vi "SET_CAPACITOR.vi"(0 "Arduino Resource in":T3, 1 "Capacitor":dbl=0.8 min=0.0 max=408.8 step=0.8 format="%.1f uF") -> (7 "Arduino Resource out":T3, 10 "error out":errorcluster)   [LabVIEW 2015]
uses:
  <vilib>/LabVIEW Interface for Arduino/Type Defs/Board Type.ctl
  <vilib>/LabVIEW Interface for Arduino/Type Defs/Connection Type.ctl
  <vilib>/LabVIEW Interface for Arduino/LabVIEW Interface for Arduino.lvlib
panel:
  in  "0, 1":i16[](array[numeric])=[1, 1, 1, 1, 1, 1, 1, 1, 1, 1, 1, 1, 1, 1, 1, 1]
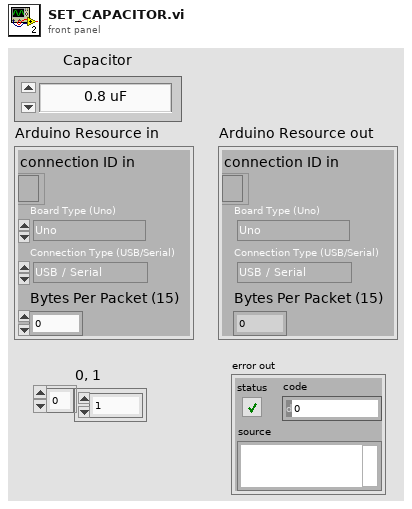
[diagram p1: front panel]
types:
  T1 = typedef "LabVIEW Interface for Arduino.lvlib/Board Type.ctl" = enum16{"Uno", "Dimuelanove w/Atmega 328", "Mega 2560"}
  T2 = typedef "LabVIEW Interface for Arduino.lvlib/Connection Type.ctl" = enum8{"USB / Serial", "XBEE", "BlueSmirf (Bluetooth)"}
  T3 = cluster{"connection ID in":refnum<k31>, "Board Type (Uno)":T1, "Connection Type (USB/Serial)":T2, "Bytes Per Packet (15)":u32}
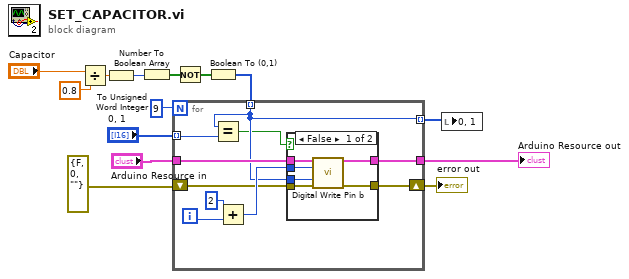
[diagram p0: block diagram]
diagram:
  n1 = Divide(x="Capacitor", y=0.8) -> (x/y=w10:dbl)
  n2 = To Unsigned Word Integer(number=w10) -> (unsigned 16bit integer=w13:u16)
  n3 = Number To Boolean Array(number=w13) -> (Boolean array=w9:bool[])
  n4 = Not(x=w9) -> (.not. x?=w8:bool[])
  n5 = Boolean To (0,1)(Boolean=w8) -> (0, 1=w12:i16[])
  n6 = for {
    N: 9 -> [_]
    tunnel: "Arduino Resource in" -> [w20]
    shift-right: [w24] -> w3
    shift-left: errorcluster {"status"=FALSE, "code"=0, "source"=""} ("error out") -> [w21]
    tunnel: [w23] -> w4
    tunnel: w12 -> [w17] mode=indexing
    tunnel: "0, 1" -> [w16] mode=indexing
    tunnel: [w17] -> w6 mode=indexing
    i -> [w19]
    n7 = Equal?(x=w17, y=w16) -> (x = y?=w15:bool)
    n8 = Add(x=2 ("y"), y=w19) -> (x+y=w22:i32)
    n9 = case shown="False" w15 {
      tunnel: [w30 w31] -> w24
      tunnel: [w29 w32] -> w23
      tunnel: w22 -> [w28 _]
      tunnel: w21 -> [w27 w31]
      tunnel: w20 -> [w26 w32]
      tunnel: w17 -> [w25 _]
      frame False {
        n10 = call "Digital Write Pin b.vi"("Arduino Resource in"=w26, "Digital I/O Pin (0)"=w28, "Value (0)"=w25, "error in"=w27) -> ("Arduino Resource out"=w29:T3, "error out"=w30:errorcluster)  [unwired: 10 in]
      }
      frame True {
      }
    }
  }
  "Arduino Resource out" <- w4
  "error out" <- w3
  n11 = local write "0, 1"(w6) -> ()
